vi "readExcel.vi"(8 "错误输入（无错误）":errorcluster, 10 "StartRow":i32=6, 11 "XlsPath":string="B:\\222.xlsx") -> (0 "错误输出":errorcluster, 2 "dataCheckOK":bool, 3 "getXYValue_string":string[][](array[string]))   [LabVIEW 2011]
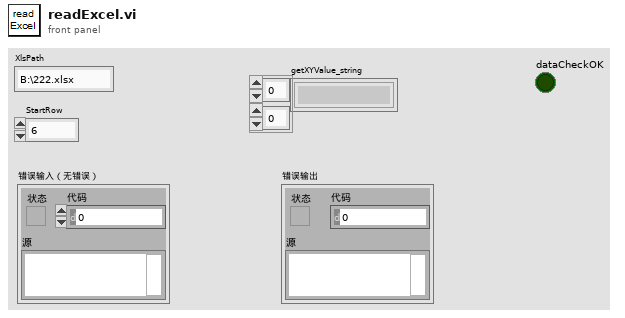
[diagram p1: front panel]
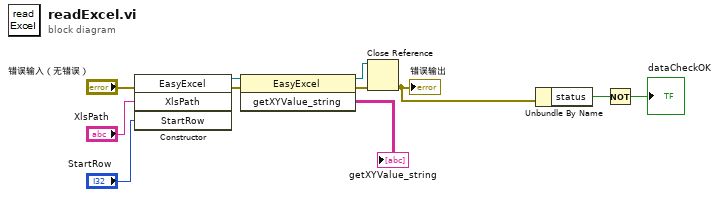
[diagram p0: block diagram]
diagram:
  n1 = constructor class="EasyExcel"(error in="错误输入（无错误）", "XlsPath"="XlsPath", "StartRow"="StartRow") -> (reference out=w11:refnum<k24>, error out=w8:errorcluster)  [unwired: 2 in, 3 out]
  n2 = invoke class="EasyExcel" method="getXYValue_string"(reference=w11, error in=w8) -> (reference out=w7:refnum<k24>, error out=w6:errorcluster, "getXYValue_string"=→"getXYValue_string":string[][])  [unwired: 1 in]
  n3 = Close Reference(reference=w7, error in (no error)=w6) -> (error out=w3:errorcluster)
  "错误输出" <- w3
  n4 = Unbundle By Name(w3) -> ("status"=w2:bool)
  n5 = Not(x=w2) -> (.not. x?=→"dataCheckOK":bool)
